vi "Generate code.vi"(1 "Terms":T1, 3 "Diagram":refnum<vi>, 5 "XRef":refnum<vi>, 6 "State In":T5) -> (0 "Generated Code?":bool, 2 "State Out":T5, 4 "Reply":string[](array[string]))   [LabVIEW 2012, in "ArrayDimension.xnode"]
uses:
  ArrayDimension.xnode
  State.ctl
  <vilib>/XNodeSupport/XNodeTermIDPairs.ctl
  <vilib>/XNodeSupport/XNodeTermIDPair.ctl
  <vilib>/XNodeSupport/XNodeTermRef.ctl
  <vilib>/XNodeSupport/XNodeString.ctl
  <vilib>/Utility/miscctls.llb/LVPositionTypeDef.ctl
  VI Scripting/Scripting Tools/Scripting Tools.lvlib
  <vilib>/XNodeSupport/NI_XNodeSupport.lvlib
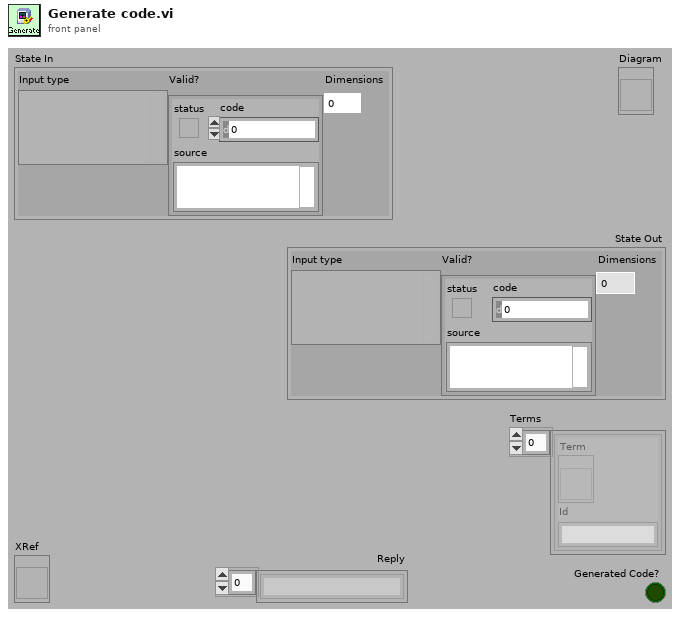
[diagram p1: front panel]
types:
  T1 = typedef "NI_XNodeSupport.lvlib/XNodeTermIDPairs.ctl" = T2[]
  T2 = typedef "NI_XNodeSupport.lvlib/XNodeTermIDPair.ctl" = cluster{"Term":T3, "Id":T4}
  T3 = typedef "NI_XNodeSupport.lvlib/XNodeTermRef.ctl" = refnum<vi>
  T4 = typedef "NI_XNodeSupport.lvlib/XNodeString.ctl" = string
  T5 = typedef "ArrayDimension.xnode/State.ctl" = cluster{"Input type":variant, "Valid?":errorcluster, "Dimensions":i32}
  T6 = typedef "LVPositionTypeDef.ctl" = cluster{"Left":i32, "Top":i32}
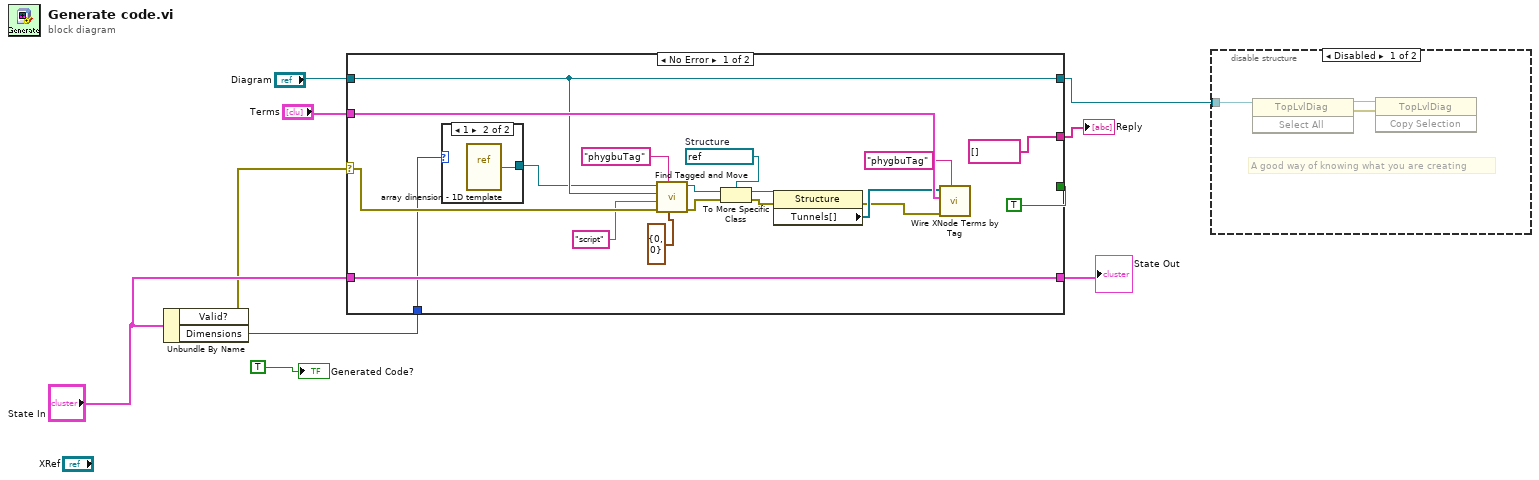
[diagram p0: block diagram]
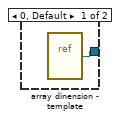
[diagram p2: hidden frame]
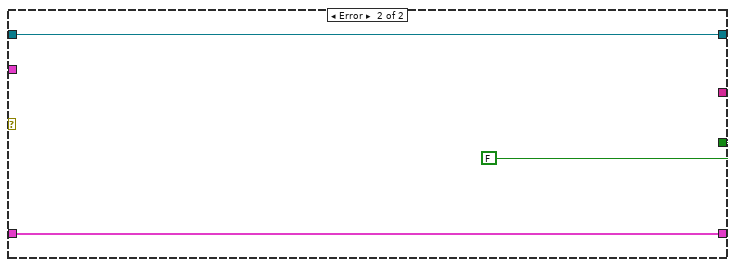
[diagram p3: hidden frame]
diagram:
  n1 = Unbundle By Name("State In") -> ("Valid?"=w2:errorcluster, "Dimensions"=w1:i32)
  n2 = case shown="No Error" w2 {
    selector: w2 -> [w21 _]
    tunnel: "State In" -> [w26 w33]
    tunnel: "Diagram" -> [w20 w31]
    tunnel: "Terms" -> [w25 _]
    tunnel: [w20 w31] -> w3
    tunnel: [string[] [] ("Reply") _] -> w4
    tunnel: [TRUE FALSE] -> _
    tunnel: [w26 w33] -> w6
    tunnel: w1 -> [w10 _]
    frame No Error {
      w23 = refnum<vi> refnum  # Structure
      n3 = case shown="1" w10 {
        tunnel: [w29 w30] -> w11
        frame 0, Default {
          n4 = vi-ref "array dinension - template.vi"() -> (w29:refnum<vi>)
        }
        frame 1 {
          n5 = vi-ref "array dinension - 1D template.vi"() -> (w30:refnum<vi>)
        }
      }
      n6 = call "Find Tagged and Move.vi"("position"=T6 {"Left"=0, "Top"=0}, "TagName"="phygbuTag", "error in"=w21, "TagValue"="script", "Destination Diagram"=w20, "VI Refnum"=w11) -> ("error out"=w15:errorcluster, "Moved Tagged object"=w16:refnum<vi>)  [unwired: 4 out]
      n7 = To More Specific Class(target class=w23, reference=w16, error in=w15) -> (specific class reference=w24:refnum<vi>, error out=w14:errorcluster)
      n8 = property class="Structure"(reference=w24, error in=w14) -> (error out=w13:errorcluster, "Tunnels[]"=w22:refnum<vi>[])  [unwired: 1 out]
      n9 = call "Wire XNode Terms by Tag.vi"("TagName"="phygbuTag", "error in (no error)"=w13, "Term Refs"=w25, "Source References"=w22) -> ()  [unwired: 8 out]
    }
    frame Error {
    }
  }
  "State Out" <- w6
  "Reply" <- w4
  n10 = disable-structure shown="Disabled" {
    disable-tunnel: w3 -> [w35 _]
    frame Disabled {
      # "A good way of knowing what you are creating"
      n11 = invoke class="TopLvlDiag" method="Select All"(reference=w35) -> (reference out=w36:refnum<vi>, error out=w34:errorcluster)  [unwired: 2 in, 1 out]
      n12 = invoke class="TopLvlDiag" method="Copy Selection"(reference=w36, error in=w34) -> ()  [unwired: 1 in, 3 out]
    }
    frame Enabled {
    }
  }
  "Generated Code?" <- TRUE
